vi "2 Ball Double Hot.vi"(1 "Run?":bool) -> (0 "Done?":bool)   [LabVIEW 2013]
uses:
  Globals/Homes.vi
  Globals/Useful Values.vi
panel:
  out "The Vision":dbl
  out "Sum":dbl
  out "Ready for Vision?":bool
  out "Side?":dbl
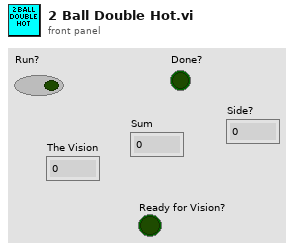
[diagram p1: front panel]
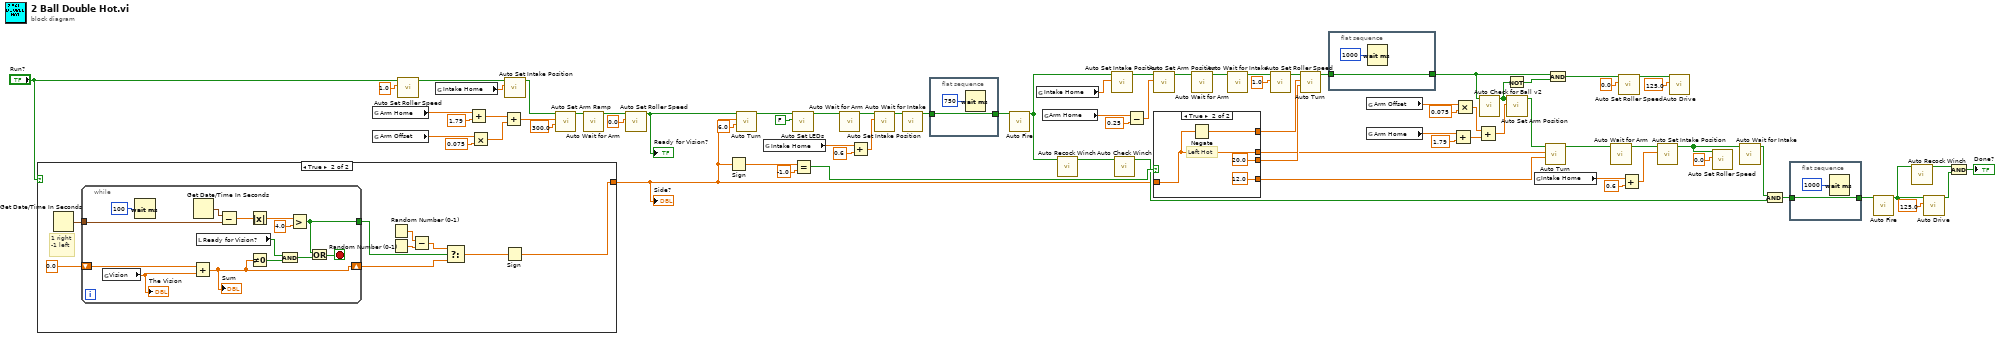
[diagram p0: block diagram]
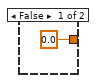
[diagram p2: hidden frame]
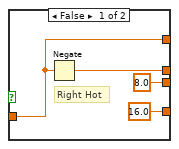
[diagram p3: hidden frame]
diagram:
  n1 = case shown="True" "Run?" {
    tunnel: [0.0 w82] -> w2
    frame False {
    }
    frame True {
      # "1 right\n-1 left"
      n2 = Get Date/Time In Seconds() -> (seconds since 1Jan1904=w89:timestamp)
      n3 = while {
        shift-right: [w100] -> w84
        shift-left: 0.0 -> [w103]
        tunnel: w89 -> [w98]
        tunnel: [w91] -> w85
        stop <- w93 stop-if-true
        n4 = global read "Useful Values.vi" "Vision"() -> (w104:dbl)
        "The Vision" <- w104
        n5 = Wait (ms)(milliseconds to wait=u32 100) -> ()  [unwired: 1 out]
        n6 = Add(x=w103, y=w104) -> (x+y=w100:dbl)
        "Sum" <- w100
        n7 = Get Date/Time In Seconds() -> (seconds since 1Jan1904=w97:timestamp)
        n8 = local read "Ready for Vision?"() -> (w101:bool)
        n9 = Subtract(x=w97, y=w98) -> (x-y=w96:dbl)
        n10 = Absolute Value(x=w96) -> (abs(x)=w95:dbl)
        n11 = Not Equal To 0?(x=w100) -> (x != 0?=w99:bool)
        n12 = And(x=w101, y=w99) -> (x .and. y?=w92:bool)
        n13 = Greater?(x=w95, y=4.0) -> (0:w91:bool)
        n14 = Or(x=w91, y=w92) -> (x .or. y?=w93:bool)
      }
      n15 = Random Number (0-1)() -> (number: 0 to 1=w86:dbl)
      n16 = Random Number (0-1)() -> (number: 0 to 1=w87:dbl)
      n17 = Subtract(x=w86, y=w87) -> (x-y=w88:dbl)
      n18 = Select(t=w88, s=w85, f=w84) -> (s? t:f=w83:dbl)
      n19 = Sign(1:w83) -> (0:w82:dbl)
    }
  }
  "Side?" <- w2
  n20 = global read "Homes.vi" "Arm Home"() -> (w76:dbl)
  n21 = global read "Useful Values.vi" "Arm Offset"() -> (w27:dbl)
  n22 = call "Auto Set Roller Speed.vi"("Value"=1.0, "Run?"="Run?") -> ("Done"=w12:bool)  [unwired: 9 in]
  n23 = global read "Homes.vi" "Intake Home"() -> (w77:dbl)
  n24 = Add(x=w76, y=1.79) -> (x+y=w24:dbl)
  n25 = Multiply(x=w27, y=0.075) -> (x*y=w25:dbl)
  n26 = Add(x=w24, y=w25) -> (x+y=w14:dbl)
  n27 = call "Auto Set Intake Position.vi"("Intake Position"=w77, "Run?"=w12) -> ("Done"=w11:bool)  [unwired: 9 in]
  n28 = call "Auto Set Arm Ramp.vi"("Time (ms)"=300.0, "Arm Position"=w14, "Run?"=w11) -> ("Done"=w4:bool)  [unwired: 8 in]
  n29 = call "Auto Wait for Arm.vi"("Run?"=w4) -> ("Done"=w5:bool)  [unwired: 10 in]
  n30 = call "Auto Set Roller Speed.vi"("Value"=0.0, "Run?"=w5) -> ("Done"=w1:bool)  [unwired: 9 in]
  "Ready for Vision?" <- w1
  n31 = Sign(1:w2) -> (0:w51:dbl)
  n32 = call "Auto Turn.vi"("Turn Amount"=6.0, "+/-?"=w2, "Run?"=w1) -> ("Done"=w80:bool)  [unwired: 8 in]
  n33 = global read "Homes.vi" "Intake Home"() -> (w75:dbl)
  n34 = call "Auto Set LEDs.vi"("LED State"=FALSE, "Run?"=w80) -> ("Done"=w79:bool)  [unwired: 9 in]
  n35 = Equal?(x=w51, y=-1.0) -> (x = y?=w49:bool)
  n36 = call "Auto Wait for Arm.vi"("Run?"=w79) -> ("Done"=w71:bool)  [unwired: 10 in]
  n37 = Add(x=w75, y=0.6) -> (x+y=w73:dbl)
  n38 = call "Auto Set Intake Position.vi"("Intake Position"=w73, "Run?"=w71) -> ("Done"=w9:bool)  [unwired: 9 in]
  n39 = call "Auto Wait for Intake.vi"("Run?"=w9) -> ("Done"=w42:bool)  [unwired: 10 in]
  n40 = flat-sequence {
    tunnel: w42 -> [w105]
    tunnel: [w105] -> w31
    frame #0 {
      n41 = Wait (ms)(milliseconds to wait=u32 750) -> ()  [unwired: 1 out]
    }
  }
  n42 = call "Auto Fire.vi"("Run?"=w31) -> ("Done"=w30:bool)  [unwired: 10 in]
  n43 = global read "Homes.vi" "Intake Home"() -> (w68:dbl)
  n44 = global read "Homes.vi" "Arm Home"() -> (w36:dbl)
  n45 = call "Auto Recock Winch.vi"("Run?"=w30) -> ("Done"=w44:bool)  [unwired: 10 in]
  n46 = call "Auto Set Intake Position.vi"("Intake Position"=w68, "Run?"=w30) -> ("Done"=w69:bool)  [unwired: 9 in]
  n47 = call "Auto Check Winch.vi"("Run?"=w44) -> ("Done"=w43:bool)  [unwired: 10 in]
  n48 = Subtract(x=w36, y=0.25) -> (x-y=w35:dbl)
  n49 = call "Auto Set Arm Position.vi"("Arm Position"=w35, "Run?"=w69) -> ("Done"=w67:bool)  [unwired: 9 in]
  n50 = case shown="True" w49 {
    tunnel: [8.0 ("Turn Amount") 20.0 ("Turn Amount")] -> w48
    tunnel: [16.0 ("Turn Amount") 12.0 ("Turn Amount")] -> w47
    tunnel: w2 -> [w108 w111]
    tunnel: [w108 w112] -> w46
    tunnel: [w107 w111] -> w45
    frame False {
      # "Right Hot"
      n51 = Negate(x=w108) -> (-x=w107:dbl)
    }
    frame True {
      # "Left Hot"
      n52 = Negate(x=w111) -> (-x=w112:dbl)
    }
  }
  n53 = call "Auto Wait for Arm.vi"("Run?"=w67) -> ("Done"=w66:bool)  [unwired: 10 in]
  n54 = call "Auto Wait for Intake.vi"("Run?"=w66) -> ("Done"=w65:bool)  [unwired: 10 in]
  n55 = call "Auto Set Roller Speed.vi"("Value"=1.0, "Run?"=w65) -> ("Done"=w63:bool)  [unwired: 9 in]
  n56 = call "Auto Turn.vi"("Turn Amount"=w48, "+/-?"=w46, "Run?"=w63) -> ("Done"=w54:bool)  [unwired: 8 in]
  n57 = flat-sequence {
    tunnel: w54 -> [w116]
    tunnel: [w116] -> w19
    frame #0 {
      n58 = Wait (ms)(milliseconds to wait=u32 1000) -> ()  [unwired: 1 out]
    }
  }
  n59 = global read "Useful Values.vi" "Arm Offset"() -> (w23:dbl)
  n60 = global read "Homes.vi" "Arm Home"() -> (w62:dbl)
  n61 = Add(x=w62, y=1.79) -> (x+y=w20:dbl)
  n62 = Multiply(x=w23, y=0.075) -> (x*y=w21:dbl)
  n63 = Add(x=w21, y=w20) -> (x+y=w15:dbl)
  n64 = call "Auto Check for Ball v2.vi"("Run?"=w19) -> ("Done"=w18:bool)  [unwired: 10 in]
  n65 = Not(x=w18) -> (.not. x?=w33:bool)
  n66 = call "Auto Set Arm Position.vi"("Arm Position"=w15, "Run?"=w18) -> ("Done"=w59:bool)  [unwired: 9 in]
  n67 = global read "Homes.vi" "Intake Home"() -> (w57:dbl)
  n68 = call "Auto Turn.vi"("Turn Amount"=w47, "+/-?"=w45, "Run?"=w59) -> ("Done"=w60:bool)  [unwired: 8 in]
  n69 = And(x=w19, y=w33) -> (x .and. y?=w32:bool)
  n70 = call "Auto Wait for Arm.vi"("Run?"=w60) -> ("Done"=w16:bool)  [unwired: 10 in]
  n71 = call "Auto Set Roller Speed.vi"("Value"=0.0, "Run?"=w32) -> ("Done"=w38:bool)  [unwired: 9 in]
  n72 = Add(x=w57, y=0.6) -> (x+y=w56:dbl)
  n73 = call "Auto Set Intake Position.vi"("Intake Position"=w56, "Run?"=w16) -> ("Done"=w53:bool)  [unwired: 9 in]
  n74 = call "Auto Drive.vi"("Amount"=125.0, "Run?"=w38) -> ()  [unwired: 9 in, 1 out]
  n75 = call "Auto Set Roller Speed.vi"("Value"=0.0, "Run?"=w53) -> ()  [unwired: 9 in, 1 out]
  n76 = call "Auto Wait for Intake.vi"("Run?"=w53) -> ("Done"=w41:bool)  [unwired: 10 in]
  n77 = And(x=w41, y=w43) -> (x .and. y?=w34:bool)
  n78 = flat-sequence {
    tunnel: w34 -> [w118]
    tunnel: [w118] -> w29
    frame #0 {
      n79 = Wait (ms)(milliseconds to wait=u32 1000) -> ()  [unwired: 1 out]
    }
  }
  n80 = call "Auto Fire.vi"("Run?"=w29) -> ("Done"=w28:bool)  [unwired: 10 in]
  n81 = call "Auto Recock Winch.vi"("Run?"=w28) -> ("Done"=w8:bool)  [unwired: 10 in]
  n82 = call "Auto Drive.vi"("Amount"=125.0, "Run?"=w28) -> ("Done"=w7:bool)  [unwired: 9 in]
  n83 = And(x=w8, y=w7) -> (x .and. y?=→"Done?":bool)
